vi "Write Plot Second Axis.vi"(4 "error in (no error)":errorcluster, 5 "Value":bool[](array[boolean]), 6 "Container State":T2, 7 "Display State In":T1) -> (0 "error out":errorcluster, 3 "Display State Out":T1)   [LabVIEW 2013, in "Configurable Buffer.xctl"]
uses:
  Configurable Buffer.xctl
  <vilib>/_xctls/Container State.ctl
  State.ctl
  <vilib>/_xctls/XControlSupport.lvlib
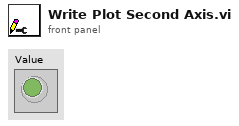
[diagram p1: front panel]
types:
  T1 = typedef "Configurable Buffer.xctl/State.ctl" = cluster{"Plot Ref":refnum<vi>, "History":i32}
  T2 = typedef "XControlSupport.lvlib/Container State.ctl" = cluster{"Indicator?":bool, "Run Mode?":bool, " Refnum":refnum<vi>}
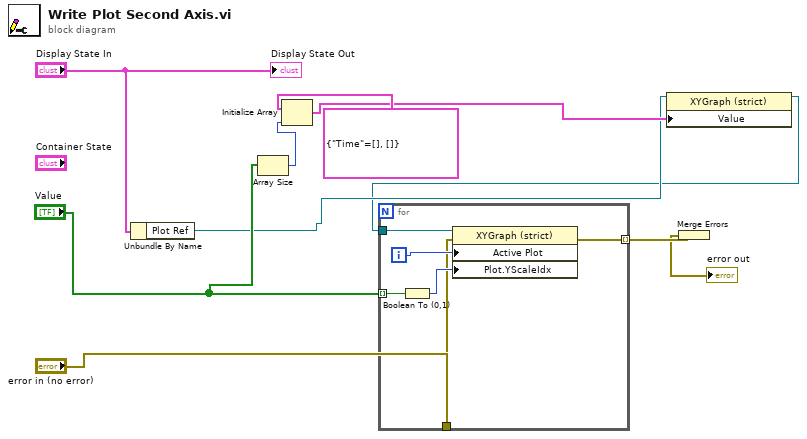
[diagram p0: block diagram]
diagram:
  n1 = Unbundle By Name("Display State In") -> ("Plot Ref"=w2:refnum<vi>)
  n2 = Array Size(array="Value") -> (size(s)=w5:i32)
  n3 = Initialize Array(cluster{"Time":timestamp[], dbl[]} {"Time"=[], []}, w5) -> (w3:cluster{"Time":timestamp[], dbl[]}[])
  n4 = property class="XYGraph (strict)"(reference=w2, "Value"=w3) -> (reference out=w1:refnum<vi>)  [unwired: 1 in, 1 out]
  n5 = for {
    tunnel: w1 -> [w16]
    tunnel: "Value" -> [w14] mode=indexing
    tunnel: [w12] -> w8 mode=indexing
    tunnel: "error in (no error)" -> [w11]
    i -> [w15]
    n6 = Boolean To (0,1)(Boolean=w14) -> (0, 1=w13:i16)
    n7 = property class="XYGraph (strict)"(reference=w16, error in=w11, "Active Plot"=w15, "Plot.YScaleIdx"=w13) -> (error out=w12:errorcluster)  [unwired: 1 out]
  }
  n8 = Merge Errors(w8) -> (→"error out":errorcluster)
  "Display State Out" <- "Display State In"
